vi "RWA_Extract Anything from String.vi"(5 "Read/Write Options (Version 1.x)":T1={"TS Fmt"="%04Y%02m%02d %02H%02M%S%25u", "Int Fmt"="%d", "Delimiter"=""}, 6 "Use Supplied (F: Use Default)":bool, 7 "Format String (%#_13g)":string="%#_13g", 8 "Error":errorcluster, 9 "Section Name":string, 10 "File String":string, 11 "Type Of Anything":variant) -> (0 "Error Out":errorcluster, 1 "Found? Out":bool, 2 "Read Failures Out":string, 3 "Anything Out":variant, 4 "All Items Found Out":bool)   [LabVIEW 2020]
doc: "This VI is designed to read data from a file written by <B>Write Anything.vi</B>. If the data type definition has changed since it was written to file, this VI will still read and fill out any elements of the cluster that have the same name. Any elements for which it cannot find a name match in the file will be supplied with their datatype's default value if Use Supplied is false. If \"Use Supplied\" is true, any elements whose name is not found in the file will use the data in the corresponding field of Type of Anything.\n\"Read/Write Options (Version 1.x)\" is used if the file at the specified Path was written with MGI Write Anything version 1.x. If the file was written with MGI Write Anything Version 2.0 or later, than the \"Read/Write Options (Version 1.x)\" input is ignored since these parameters are stored in the data file itself.\nAuthored by Robert C. Mortensen\nsupport@mooregoodideas.com\nwww.mooregoodideas.com\n\nCopyright (c) 2010, Moore Good Ideas, Inc.\n\nAll rights reserved.\n\nRedistribution and use in source and binary forms, with or without modification, are permitted provided that the following conditions are met:\n\n * Redistributions of source code must retain the above copyright notice, this list of conditions and the following disclaimer.\n * Redistributions in binary form must reproduce the above copyright notice, this list of conditions and the following disclaimer in the documentation and/or other materials provided with the distribution.\n * Neither the name of Moore Good Ideas, Inc. nor the names of its contributors may be used to endorse or promote products derived from this software without specific prior written permission.\n\nTHIS SOFTWARE IS PROVIDED BY THE COPYRIGHT HOLDERS AND CONTRIBUTORS \"AS IS\" AND ANY EXPRESS OR IMPLIED WARRANTIES, INCLUDING, BUT NOT LIMITED TO, THE IMPLIED WARRANTIES OF MERCHANTABILITY AND FITNESS FOR A PARTICULAR PURPOSE ARE DISCLAIMED. IN NO EVENT SHALL THE COPYRIGHT OWNER OR CONTRIBUTORS BE LIABLE FOR ANY DIRECT, INDIRECT, INCIDENTAL, SPECIAL, EXEMPLARY, OR CONSEQUENTIAL DAMAGES (INCLUDING, BUT NOT LIMITED TO, PROCUREMENT OF SUBSTITUTE GOODS OR SERVICES; LOSS OF USE, DATA, OR PROFITS; OR BUSINESS INTERRUPTION) HOWEVER CAUSED AND ON ANY THEORY OF LIABILITY, WHETHER IN CONTRACT, STRICT LIABILITY, OR TORT (INCLUDING NEGLIGENCE OR OTHERWISE) ARISING IN ANY WAY OUT OF THE USE OF THIS SOFTWARE, EVEN IF ADVISED OF THE POSSIBILITY OF SUCH DAMAGE."
uses:
  MGI RWA Options Cluster.ctl
  <vilib>/Utility/Data Type/NI_Data Type.lvlib
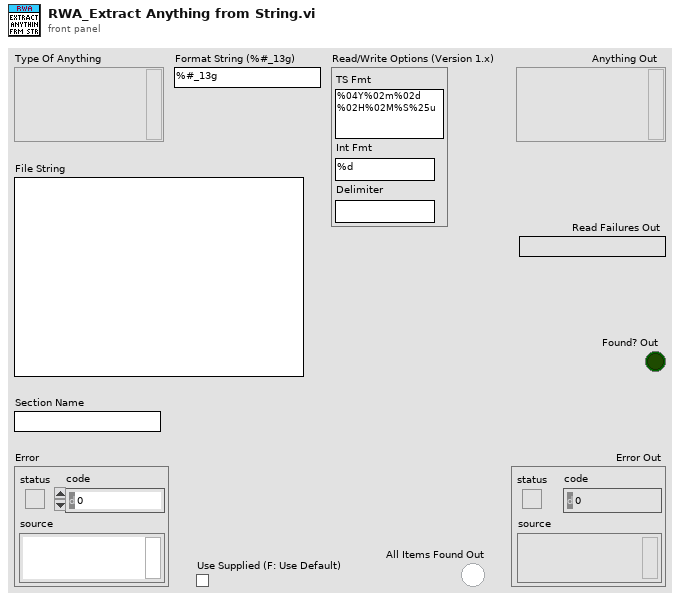
[diagram p1: front panel]
types:
  T1 = typedef "MGI RWA Options Cluster.ctl" = cluster{"TS Fmt":string, "Int Fmt":string, "Delimiter":string}
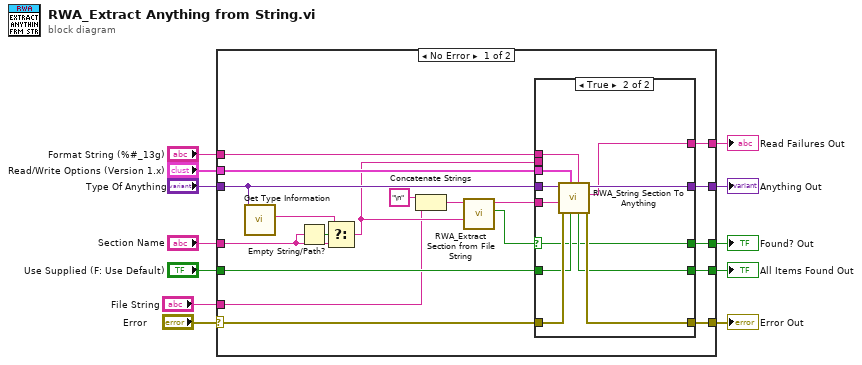
[diagram p0: block diagram]
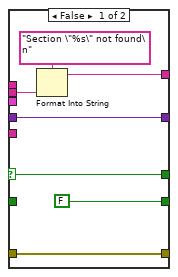
[diagram p2: hidden frame]
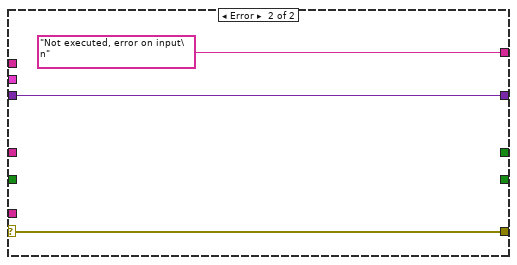
[diagram p3: hidden frame]
diagram:
  n1 = case shown="No Error" "Error" {
    selector: "Error" -> [w16 w52]
    tunnel: [w31 w52] -> w12
    tunnel: [w30 w51] -> w11
    tunnel: [w13 _] -> w10
    tunnel: "Section Name" -> [w28 _]
    tunnel: "Type Of Anything" -> [w26 w51]
    tunnel: "Read/Write Options (Version 1.x)" -> [w25 _]
    tunnel: "Format String (%#_13g)" -> [w24 _]
    tunnel: "Use Supplied (F: Use Default)" -> [w23 _]
    tunnel: [w22 "Not executed, error on input\n"] -> w3
    tunnel: [w21 _] -> w2
    tunnel: "File String" -> [w15 _]
    frame No Error {
      n2 = call <vilib>:"Get Type Information.vi"("variant"=w26) -> ("name"=w27:string)  [unwired: 6 in, 4 out]
      n3 = Empty String/Path?(string/path=w28) -> (empty?=w29:bool)
      n4 = Select(t=w27, s=w29, f=w28) -> (s? t:f=w17:string)
      n5 = Concatenate Strings("\n" ("string"), w15) -> (w20:string)
      n6 = call "RWA_Extract Section from File String.vi"("Section Name"=w17, "String"=w20) -> ("Found? Out"=w14:bool, "String Out"=w18:string)  [unwired: 8 in]
      n7 = case shown="True" w14 {
        selector: w14 -> [w32 w39]
        tunnel: [w37 w49] -> w31
        tunnel: [w38 w48] -> w30
        tunnel: w26 -> [w38 w40]
        tunnel: w16 -> [w37 w47]
        tunnel: w25 -> [_ w41]
        tunnel: w18 -> [_ w46]
        tunnel: w24 -> [_ w42]
        tunnel: w23 -> [_ w43]
        tunnel: [w35 w45] -> w22
        tunnel: w17 -> [w36 _]
        tunnel: [FALSE ("All Items found") w44] -> w21
        tunnel: [w32 w39] -> w13
        frame False {
          n8 = Format Into String(format string="Section \"%s\" not found\n", w36) -> (resulting string=w35:string)  [unwired: 2 in, 1 out]
        }
        frame True {
          n9 = call "RWA_String Section To Anything.vi"("Format String (%#_13g)"=w42, "Use Supplied"=w43, "Read/Write Options"=w41, "Error"=w47, "String Section"=w46, "Type Of Anything"=w40) -> ("Error Out"=w49:errorcluster, "Read Failures Out"=w45:string, "Type Of Anything Out"=w48:variant, "All Items Found Out"=w44:bool)  [unwired: 2 in]
        }
      }
    }
    frame Error {
    }
  }
  "Error Out" <- w12
  "Anything Out" <- w11
  "Found? Out" <- w10
  "Read Failures Out" <- w3
  "All Items Found Out" <- w2
